vi "swervecalculations.vi"(9 "z":dbl, 10 "y":dbl, 11 "x":dbl) -> (0 "4 ang":dbl, 1 "3 ang":dbl, 2 "2 ang":dbl, 3 "1 ang":dbl, 4 "2 speed":dbl, 5 "1 speed":dbl, 7 "3 speed":dbl)   [LabVIEW 2017]
panel:
  out "4 speed":dbl
  out "d":dbl
  out "c":dbl
  out "b":dbl
  out "a":dbl
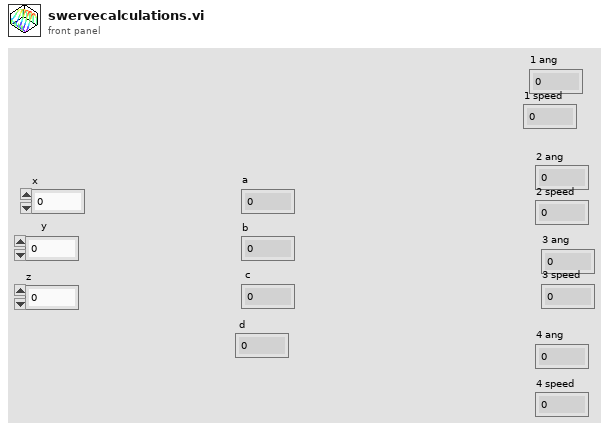
[diagram p1: front panel]
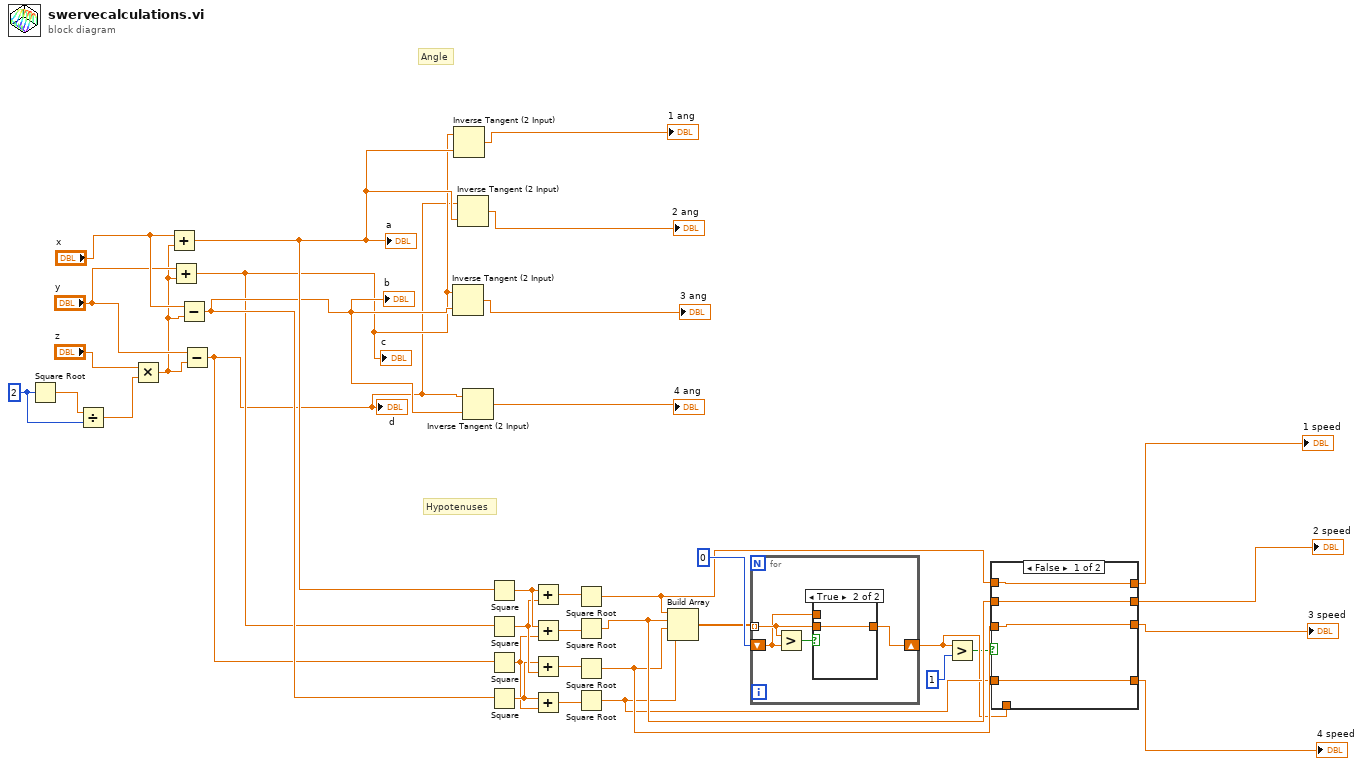
[diagram p0: block diagram]
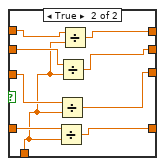
[diagram p2: hidden frame]
diagram:
  w36 = 2
  # "Hypotenuses"
  # "Angle"
  n1 = Square Root(x=w36) -> (sqrt(x)=w35:dbl)
  n2 = Divide(x=w35, y=w36) -> (x/y=w33:dbl)
  n3 = Multiply(x="z", y=w33) -> (x*y=w30:dbl)
  n4 = Add(x="x", y=w30) -> (x+y=w25:dbl)
  "a" <- w25
  n5 = Add(x="y", y=w30) -> (x+y=w23:dbl)
  "c" <- w23
  n6 = Subtract(x="x", y=w30) -> (x-y=w24:dbl)
  "b" <- w24
  n7 = Subtract(x="y", y=w30) -> (x-y=w22:dbl)
  "d" <- w22
  n8 = Inverse Tangent (2 Input)(1:w24, 2:w23) -> (0:→"3 ang":dbl)
  n9 = Inverse Tangent (2 Input)(1:w25, 2:w23) -> (0:→"1 ang":dbl)
  n10 = Inverse Tangent (2 Input)(1:w25, 2:w22) -> (0:→"2 ang":dbl)
  n11 = Inverse Tangent (2 Input)(1:w24, 2:w22) -> (0:→"4 ang":dbl)
  n12 = Square(x=w25) -> (x^2=w21:dbl)
  n13 = Square(x=w23) -> (x^2=w20:dbl)
  n14 = Square(x=w22) -> (x^2=w18:dbl)
  n15 = Square(x=w24) -> (x^2=w19:dbl)
  n16 = Add(x=w21, y=w20) -> (x+y=w14:dbl)
  n17 = Add(x=w21, y=w18) -> (x+y=w15:dbl)
  n18 = Add(x=w19, y=w20) -> (x+y=w16:dbl)
  n19 = Add(x=w19, y=w18) -> (x+y=w17:dbl)
  n20 = Square Root(x=w14) -> (sqrt(x)=w10:dbl)
  n21 = Square Root(x=w15) -> (sqrt(x)=w9:dbl)
  n22 = Square Root(x=w16) -> (sqrt(x)=w8:dbl)
  n23 = Square Root(x=w17) -> (sqrt(x)=w7:dbl)
  n24 = Build Array(w10, w9, w8, w7) -> (w12:dbl[])
  n25 = for {
    shift-right: [w38] -> w6
    shift-left: 0 -> [w37]
    tunnel: w12 -> [w39] mode=indexing
    n26 = Greater?(x=w39, y=w37) -> (0:w40:bool)
    n27 = case shown="True" w40 {
      tunnel: w39 -> [_ w42]
      tunnel: [w41 w42] -> w38
      tunnel: w37 -> [w41 _]
      frame False {
      }
      frame True {
      }
    }
  }
  n28 = Greater?(x=w6, y=1) -> (0:w1:bool)
  n29 = case shown="False" w1 {
    tunnel: w10 -> [w46 w55]
    tunnel: w9 -> [w45 w54]
    tunnel: w8 -> [w44 w53]
    tunnel: w7 -> [w43 w52]
    tunnel: [w46 w47] -> w5
    tunnel: [w45 w48] -> w4
    tunnel: [w44 w49] -> w3
    tunnel: [w43 w50] -> w2
    tunnel: w6 -> [_ w51]
    frame False {
    }
    frame True {
      n30 = Divide(x=w52, y=w51) -> (x/y=w50:dbl)
      n31 = Divide(x=w53, y=w51) -> (x/y=w49:dbl)
      n32 = Divide(x=w54, y=w51) -> (x/y=w48:dbl)
      n33 = Divide(x=w55, y=w51) -> (x/y=w47:dbl)
    }
  }
  "1 speed" <- w5
  "2 speed" <- w4
  "3 speed" <- w3
  "4 speed" <- w2
